vi "TDT-zBusTrig.vi"(4 "error in (no error)":errorcluster) -> (0 "error out":errorcluster)   [LabVIEW 2020]
doc: "Sends <B>Start</B> notifier to DAQ thread to begin measurement."
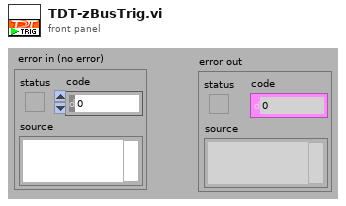
[diagram p1: front panel]
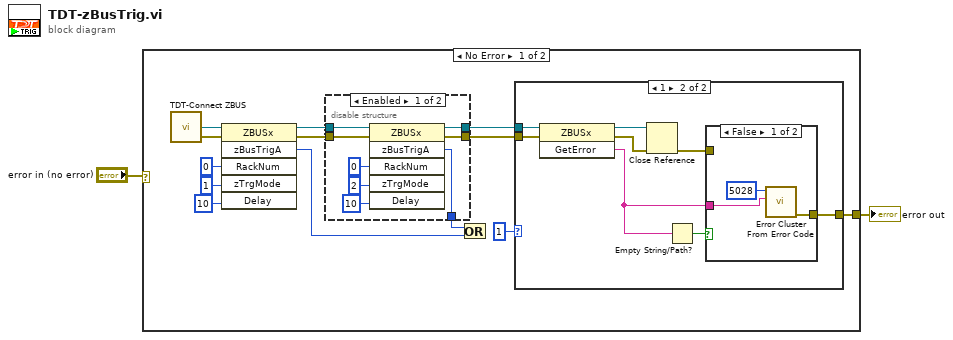
[diagram p0: block diagram]
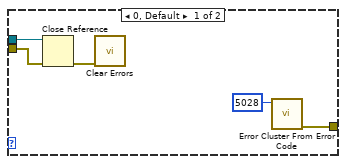
[diagram p3: hidden frame]
diagram:
  n1 = case shown="No Error" "error in (no error)" {
    selector: "error in (no error)" -> [_ w43]
    tunnel: [w9 w43] -> w1
    frame No Error {
      n2 = call "TDT-Connect ZBUS.vi"() -> ("ZBUSx"=w4:refnum<k7>, "error out"=w3:errorcluster)  [unwired: 14 in]
      n3 = invoke class="ZBUSx" method="zBusTrigA"(reference=w4, error in=w3, "RackNum"=0, "zTrgMode"=1, "Delay"=10) -> (reference out=w12:refnum<k7>, error out=w11:errorcluster, "zBusTrigA"=w10:i32)  [unwired: 1 in, 3 out]
      n4 = disable-structure shown="Enabled" {
        disable-tunnel: w12 -> [w23 w25]
        disable-tunnel: w11 -> [w22 w24]
        disable-tunnel: [w21 w24] -> w8
        disable-tunnel: [w20 w25] -> w7
        disable-tunnel: [w19 _] -> w5
        frame Enabled {
          n5 = invoke class="ZBUSx" method="zBusTrigA"(reference=w23, error in=w22, "RackNum"=0, "zTrgMode"=2, "Delay"=10) -> (reference out=w20:refnum<k7>, error out=w21:errorcluster, "zBusTrigA"=w19:i32)  [unwired: 1 in, 3 out]
        }
        frame Disabled {
        }
      }
      n6 = Or(x=w5, y=w10) -> ()  [unwired: 1 out]
      n7 = case shown="1" 1 {
        tunnel: [w29 w34] -> w9
        tunnel: w8 -> [w27 w38]
        tunnel: w7 -> [w28 w37]
        frame 0, Default {
          n8 = Close Reference(reference=w28, error in (no error)=w27) -> (error out=w26:errorcluster)
          n9 = call <vilib>:"Clear Errors.vi"("error in (no error)"=w26) -> ()  [unwired: 5 in, 2 out]
          n10 = call <vilib>:"Error Cluster From Error Code.vi"("error code (0)"=5028) -> ("error out"=w29:errorcluster)  [unwired: 8 in]
        }
        frame 1 {
          n11 = invoke class="ZBUSx" method="GetError"(reference=w37, error in=w38) -> (reference out=w33:refnum<k7>, error out=w32:errorcluster, "GetError"=w35:string)  [unwired: 1 in]
          n12 = Close Reference(reference=w33, error in (no error)=w32) -> (error out=w31:errorcluster)
          n13 = Empty String/Path?(string/path=w35) -> (empty?=w36:bool)
          n14 = case shown="False" w36 {
            tunnel: w35 -> [w40 _]
            tunnel: [w39 w42] -> w34
            tunnel: w31 -> [_ w42]
            frame False {
              n15 = call <vilib>:"Error Cluster From Error Code.vi"("error message (\"\")"=w40, "error code (0)"=5028) -> ("error out"=w39:errorcluster)  [unwired: 7 in]
            }
            frame True {
            }
          }
        }
      }
    }
    frame Error {
    }
  }
  "error out" <- w1
